vi "Get Tag LUT.vi"(8 "error in (no error)":errorcluster) -> (0 "error out":errorcluster, 3 "Tag LUT Out":refnum<data-value>)   [LabVIEW 2020, in "Tag Engine Core.lvlib" / "Tag Core.lvclass"]
doc: "_SubVI_"
uses:
  Tag Core.lvclass
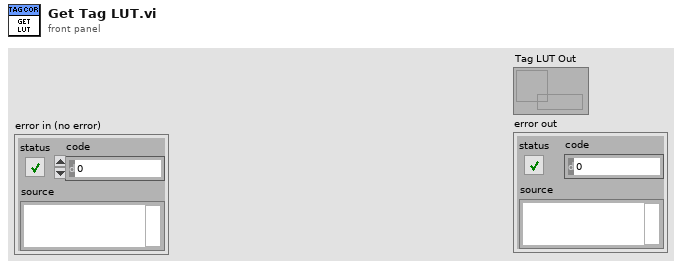
[diagram p1: front panel]
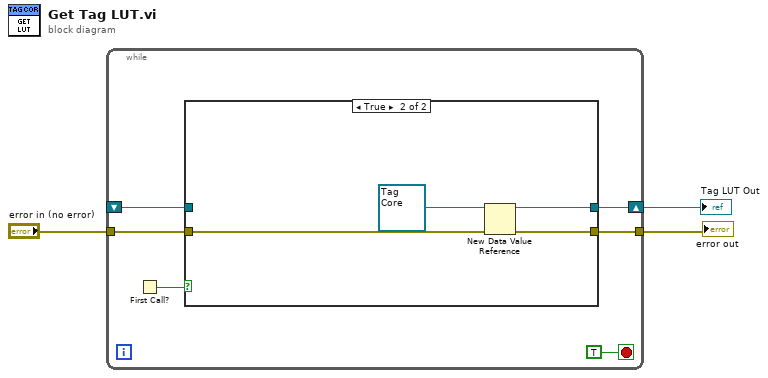
[diagram p0: block diagram]
diagram:
  n1 = while {
    shift-right: [w8] -> w3
    shift-left: _ -> [w7]
    tunnel: [w5] -> w2
    tunnel: "error in (no error)" -> [w4]
    stop <- TRUE stop-if-true
    n2 = First Call?() -> (First Call?: T/F=w9:bool)
    n3 = case shown="True" w9 {
      tunnel: [w11 w15] -> w8
      tunnel: w7 -> [w11 _]
      tunnel: [w10 w14] -> w5
      tunnel: w4 -> [w10 w13]
      frame False {
      }
      frame True {
        n4 = New Data Value Reference(data value=refnum<class "Tag Core.lvclass"> refnum ("CVT Core.lvclass"), error in=w13) -> (data value reference=w15:refnum<data-value>, error out=w14:errorcluster)
      }
    }
  }
  "Tag LUT Out" <- w3
  "error out" <- w2
